vi "Temp Sensor.vi"() -> (2 "Temperature (°C)":dbl)   [LabVIEW 2014]
uses:
  Global Stop TempSensor.vi
panel:
  in  "stop":bool
  in  "Current Temp (°C)":dbl(slide)=70.0 scale=0.0..100.0
  in  "High Limit (°C)":dbl=70.0
  out "Warning Txt":string
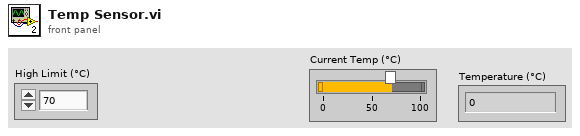
[diagram p1: front panel]
types:
  T1 = enum32{"Invalid", "Standard", "Closed", "Hidden", "Minimized", "Maximized"}
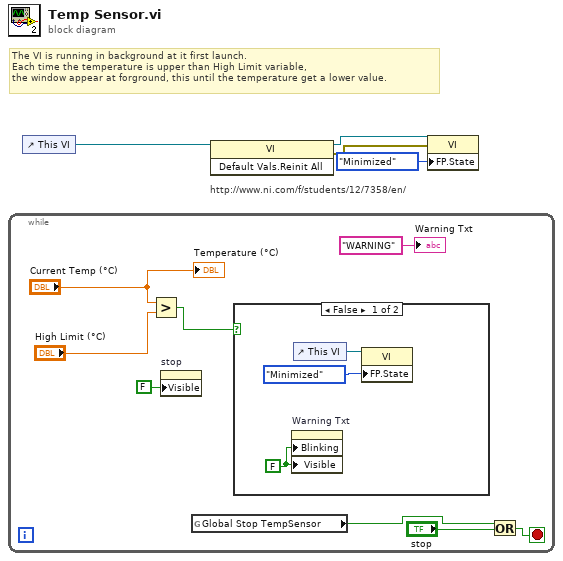
[diagram p0: block diagram]
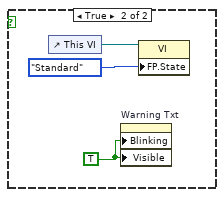
[diagram p2: hidden frame]
diagram:
  # "http://www.ni.com/f/students/12/7358/en/"
  # "The VI is running in background at it first launch.\nEach time the temperature is upper than High Limit variable,\nthe window appear at forground, this until the temperature get a lower value."
  n1 = while {
    stop <- w7 stop-if-true
    n2 = Greater?(x="Current Temp (°C)", y="High Limit (°C)") -> (0:w11:bool)
    n3 = property on="stop" class="Bool"("Visible"=FALSE) -> ()  [unwired: 2 in, 2 out]
    n4 = global read "Global Stop TempSensor.vi" "Global Stop TempSensor"() -> (w5:bool)
    n5 = case shown="False" w11 {
      frame False {
        w15 = FALSE
        n6 = property on="Warning Txt" class="Str"("Blinking"=w15, "Visible"=w15) -> ()  [unwired: 2 in, 2 out]
        n7 = control-ref of="This VI"() -> (w13:refnum<vi>)
        n8 = property class="VI"(reference=w13, "FP.State"=T1."Minimized" ("Front Panel Window:State")) -> ()  [unwired: 1 in, 2 out]
      }
      frame True {
        w18 = TRUE
        n9 = control-ref of="This VI"() -> (w16:refnum<vi>)
        n10 = property on="Warning Txt" class="Str"("Blinking"=w18, "Visible"=w18) -> ()  [unwired: 2 in, 2 out]
        n11 = property class="VI"(reference=w16, "FP.State"=T1."Standard" ("Front Panel Window:State")) -> ()  [unwired: 1 in, 2 out]
      }
    }
    n12 = Or(x=w5, y="stop") -> (x .or. y?=w7:bool)
    "Temperature (°C)" <- "Current Temp (°C)"
    "Warning Txt" <- "WARNING" ("Warning Txt")
  }
  n13 = control-ref of="This VI"() -> (w4:refnum<vi>)
  n14 = invoke class="VI" method="Default Vals.Reinit All"(reference=w4) -> (reference out=w3:refnum<vi>, error out=w2:errorcluster)  [unwired: 2 in, 1 out]
  n15 = property class="VI"(reference=w3, error in=w2, "FP.State"=T1."Minimized" ("Front Panel Window:State")) -> ()  [unwired: 2 out]
